vi "Get List Information.vi"(8 "List Selection":string, 9 "DQMH Scan Info":T3, 10 "References Map":map{string, refnum<vi>}(c390), 11 "Tree Map":T5) -> (0 "Documentation":T2, 1 "Clon?":bool, 2 "Vi out":refnum<vi>, 3 "Module type":T1, 4 "VI Connector Pane":picture, 5 "DQMH Lib":refnum<vi>, 6 "Broadcast?":bool)   [LabVIEW 2019, in "Panther Dashboard.lvlib"]
uses:
  Panther Dashboard.lvlib
  <vilib>/National Instruments/Tree Map/Tree Map Data.ctl
  DQMH Modules Info--cluster.ctl
  Module type--enum.ctl
  Project References--cluster.ctl
  Documentation--cluster.ctl
  <vilib>/National Instruments/Tree Map/Tree Map.lvlib
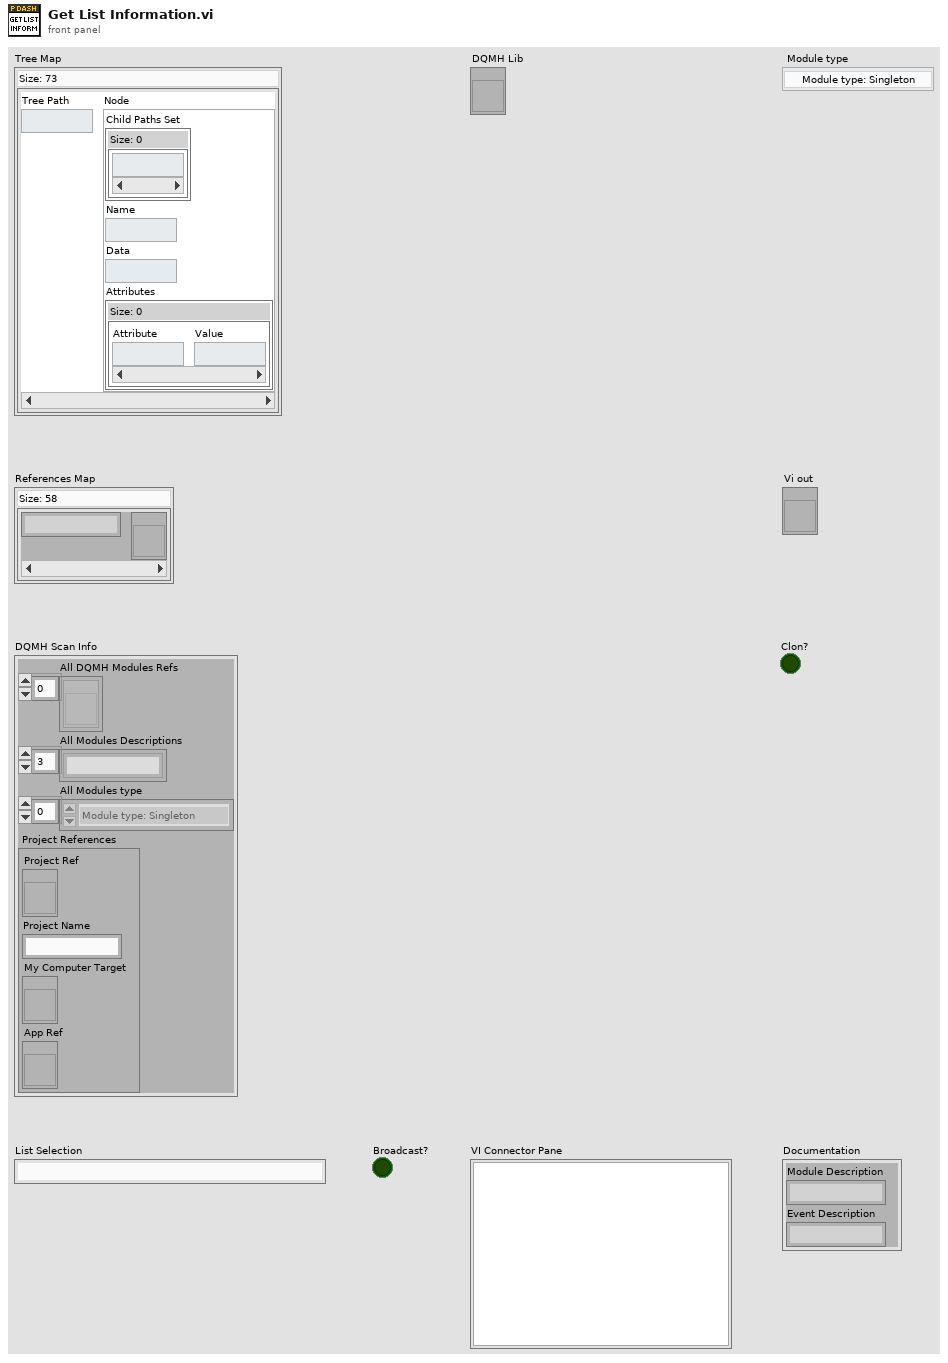
[diagram p1: front panel]
types:
  T1 = typedef "Panther Dashboard.lvlib/Module type--enum.ctl" = enum16{"Module type: Singleton", "Module type: Cloneable"}
  T2 = typedef "Panther Dashboard.lvlib/Documentation--cluster.ctl" = cluster{"Module Description":string, "Event Description":string}
  T3 = typedef "Panther Dashboard.lvlib/DQMH Modules Info--cluster.ctl" = cluster{"All DQMH Modules Refs":refnum<vi>[], "All Modules Descriptions":string[], "All Modules type":T1[], "Project References":T4}
  T4 = typedef "Panther Dashboard.lvlib/Project References--cluster.ctl" = cluster{"Project Ref":refnum<vi>, "Project Name":string, "My Computer Target":refnum<vi>, "App Ref":refnum<vi>}
  T5 = typedef "Tree Map.lvlib/Tree Map Data.ctl" = map{string, cluster{"Child Paths Set":set{string}, "Name":string, "Data":string, "Attributes":map{string, string}}}
  T6 = cluster{"Child Paths Set":set{string}, "Name":string, "Data":string, "Attributes":map{string, string}}
  T7 = cluster{"Description":string, "VI Description":string}
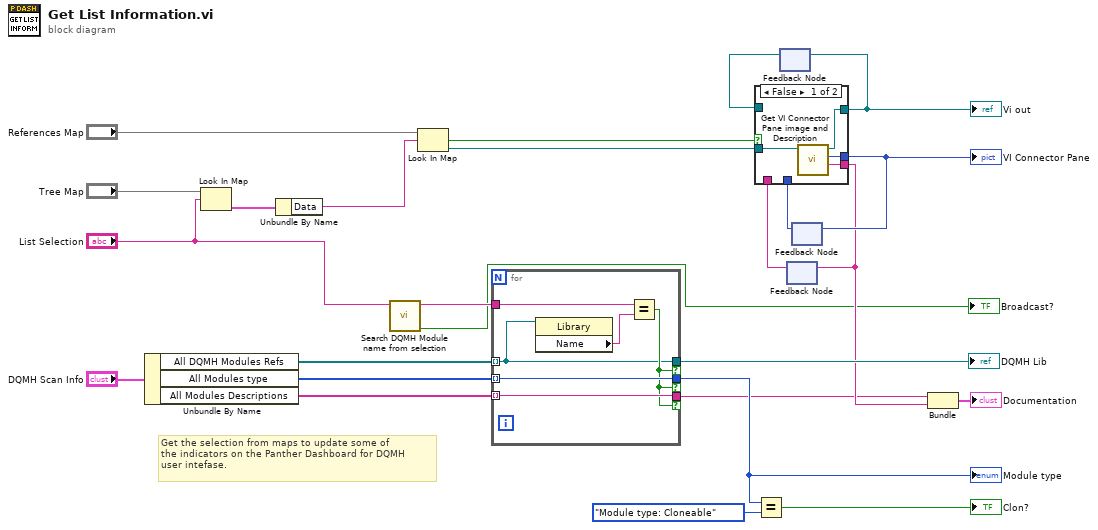
[diagram p0: block diagram]
diagram:
  # "Get the selection from maps to update some of\nthe indicators on the Panther Dashboard for DQMH \nuser intefase."
  n1 = Unbundle By Name("DQMH Scan Info") -> ("All DQMH Modules Refs"=w17:refnum<vi>[], "All Modules type"=w16:T1[], "All Modules Descriptions"=w15:string[])
  n2 = Look In Map(map="Tree Map", key="List Selection") -> (value=w24:T6)  [unwired: 1 in, 1 out]
  n3 = Unbundle By Name(w24) -> ("Data"=w20:string)
  n4 = call "Search DQMH Module name from selection.vi"("Search Module Name"="List Selection") -> ("Broadcast?"=→"Broadcast?":bool, "Module Name"=w14:string)  [unwired: 9 in]
  n5 = Look In Map(map="References Map", key=w20) -> (key not found?=w21:bool, value=w19:refnum<vi>)  [unwired: 1 in]
  n6 = for {
    tunnel: w17 -> [w27] mode=indexing
    tunnel: w16 -> [w30] mode=indexing
    tunnel: w15 -> [w29] mode=indexing
    tunnel: w14 -> [w31]
    tunnel: [w27] -> w12 if=w28
    tunnel: [w30] -> w5 if=w28
    tunnel: [w29] -> w1 if=w28
    n7 = property class="Library"(reference=w27) -> ("Name"=w26:string)  [unwired: 1 in, 2 out]
    n8 = Equal?(x=w31, y=w26) -> (x = y?=w28:bool)
  }
  "DQMH Lib" <- w12
  "Module type" <- w5
  n9 = Equal?(x=w5, y=Module_type--enum."Module type: Cloneable") -> (x = y?=→"Clon?":bool)
  n10 = feedback #1() -> (w10:refnum<vi>)  [unwired: 1 in]
  n11 = feedback #2() -> (w6:string)  [unwired: 1 in]
  n12 = feedback #3() -> (w8:picture)  [unwired: 1 in]
  n13 = case shown="False" w21 {
    tunnel: w19 -> [w35 _]
    tunnel: [w34 w37] -> w9
    tunnel: [w33 w38] -> w11
    tunnel: [w32 w36] -> w7
    tunnel: w10 -> [_ w38]
    tunnel: w8 -> [_ w37]
    tunnel: w6 -> [_ w36]
    frame False {
      n14 = call "Get VI Connector Pane image and Description.vi"("VI in"=w35) -> ("VI Description"=w32:string, "VI Connector Pane"=w34:picture, "Vi out"=w33:refnum<vi>)  [unwired: 7 in, 1 out]
    }
    frame True {
    }
  }
  "VI Connector Pane" <- w9
  "Vi out" <- w11
  n15 = feedback-in #1(w11) -> ()
  n16 = feedback-in #2(w7) -> ()
  n17 = feedback-in #3(w9) -> ()
  n18 = Bundle("Description"=w1, "VI Description"=w7) -> (→"Documentation":T7)  [unwired: 1 in]
